vi "MAVLink RAW IMU.vi"(7 "FGV Method":T2, 11 "Raw IMU":T1) -> (3 "Raw IMU out":T1)   [LabVIEW 2014]
uses:
  Controls/FGV Methods.ctl
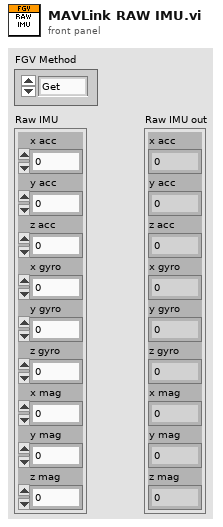
[diagram p1: front panel]
types:
  T1 = cluster{"x acc":i16, "y acc":i16, "z acc":i16, "x gyro":i16, "y gyro":i16, "z gyro":i16, "x mag":i16, "y mag":i16, "z mag":i16}
  T2 = typedef "FGV Methods.ctl" = enum16{"Get", "Set"}
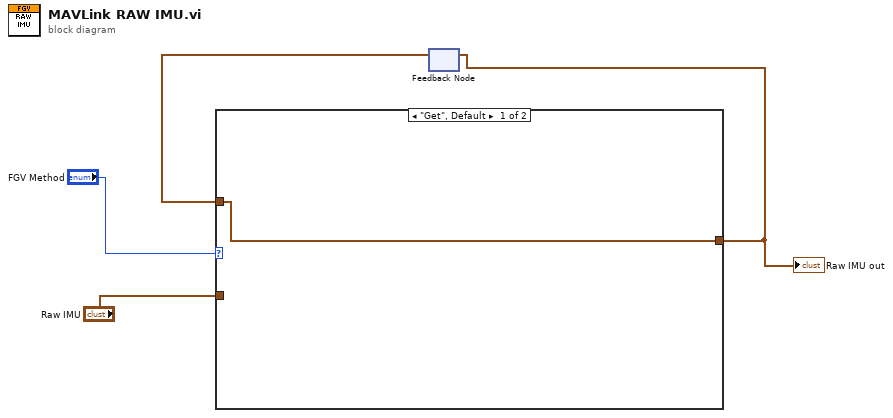
[diagram p0: block diagram]
diagram:
  n1 = feedback #1() -> (w2:T1)  [unwired: 1 in]
  n2 = case shown="\"Get\", Default" "FGV Method" {
    tunnel: "Raw IMU" -> [_ w6]
    tunnel: [w5 w6] -> w3
    tunnel: w2 -> [w5 _]
    frame "Get", Default {
    }
    frame "Set" {
    }
  }
  "Raw IMU out" <- w3
  n3 = feedback-in #1(w3) -> ()
